vi "Main UI.vi"(11 "FormulaLV App in":refnum<class "FormulaG App.lvclass">) -> ()   [LabVIEW 2024, in "FormulaG.lvlib" / "FormulaG App.lvclass"]
uses:
  FormulaG App.lvclass
  FormulaG-Common/Camera.ctl
  <vilib>/sklein/WebView2/Webview2 Control/WebView2 Control.xctl
  UI State.ctl
  FormulaG App.lvclass/FormulaG App.ctl
  FormulaG-Common/UI Options.ctl
  State Update.ctl
  FormulaG-Common/Car State.ctl
  FormulaG-Common/Ranges.ctl
  FormulaG-Common/Car Info.ctl
  FormulaG-Common/Car Control.ctl
  FormulaG-Common/FormulaG-Common.lvlib
  FormulaG API/FormulaG API.lvclass
  <vilib>/IlluminatedG/IG GodotServer/GodotLV/GodotServer/GodotServer.lvclass
  Pause Cmd/Pause Cmd.lvclass
  Select Cam Cmd/Select Cam Cmd.lvclass
  UI Options Cmd/UI Options Cmd.lvclass
  Reset Cmd/Reset Cmd.lvclass
  <vilib>/IlluminatedG/IG OBS API/obs-websocket/OBS/OBS.lvclass
panel:
  out "UI Cover":string="\n\n\n\n\n\n\n\n\n\n\n\n\n\n\n\n\nWaiting for connection to game engine..."
  out "Fastest Lap":i32
  out "Fastest Lap Time":dbl format="%<%M:%S%3u>t"
  out "Lap":u8
  out "Update Rate":dbl format="%.2f"
  out "Web":string(xcontrol)
  out "Throttle":sgl(slide) scale=0.0..1.0
  out "Speed":sgl(knob) scale=0.0..10.0
  in  "Clear Map":bool
  out "Last Lap":dbl format="%<%M:%S%3u>t"
  out "Current Lap":dbl format="%<%M:%S%3u>t"
  out "XY Graph":cluster{dbl[], dbl[]}[](graph)
  in  "Pause":bool
  out "Chart":dbl[][](graph)
  in  "Camera":T1
  in  "Reset":bool
  out "Steering":sgl(knob) scale=-1.0..1.0
  out "Connected":bool
  in  "Show Range Lines":bool
  # "Map"
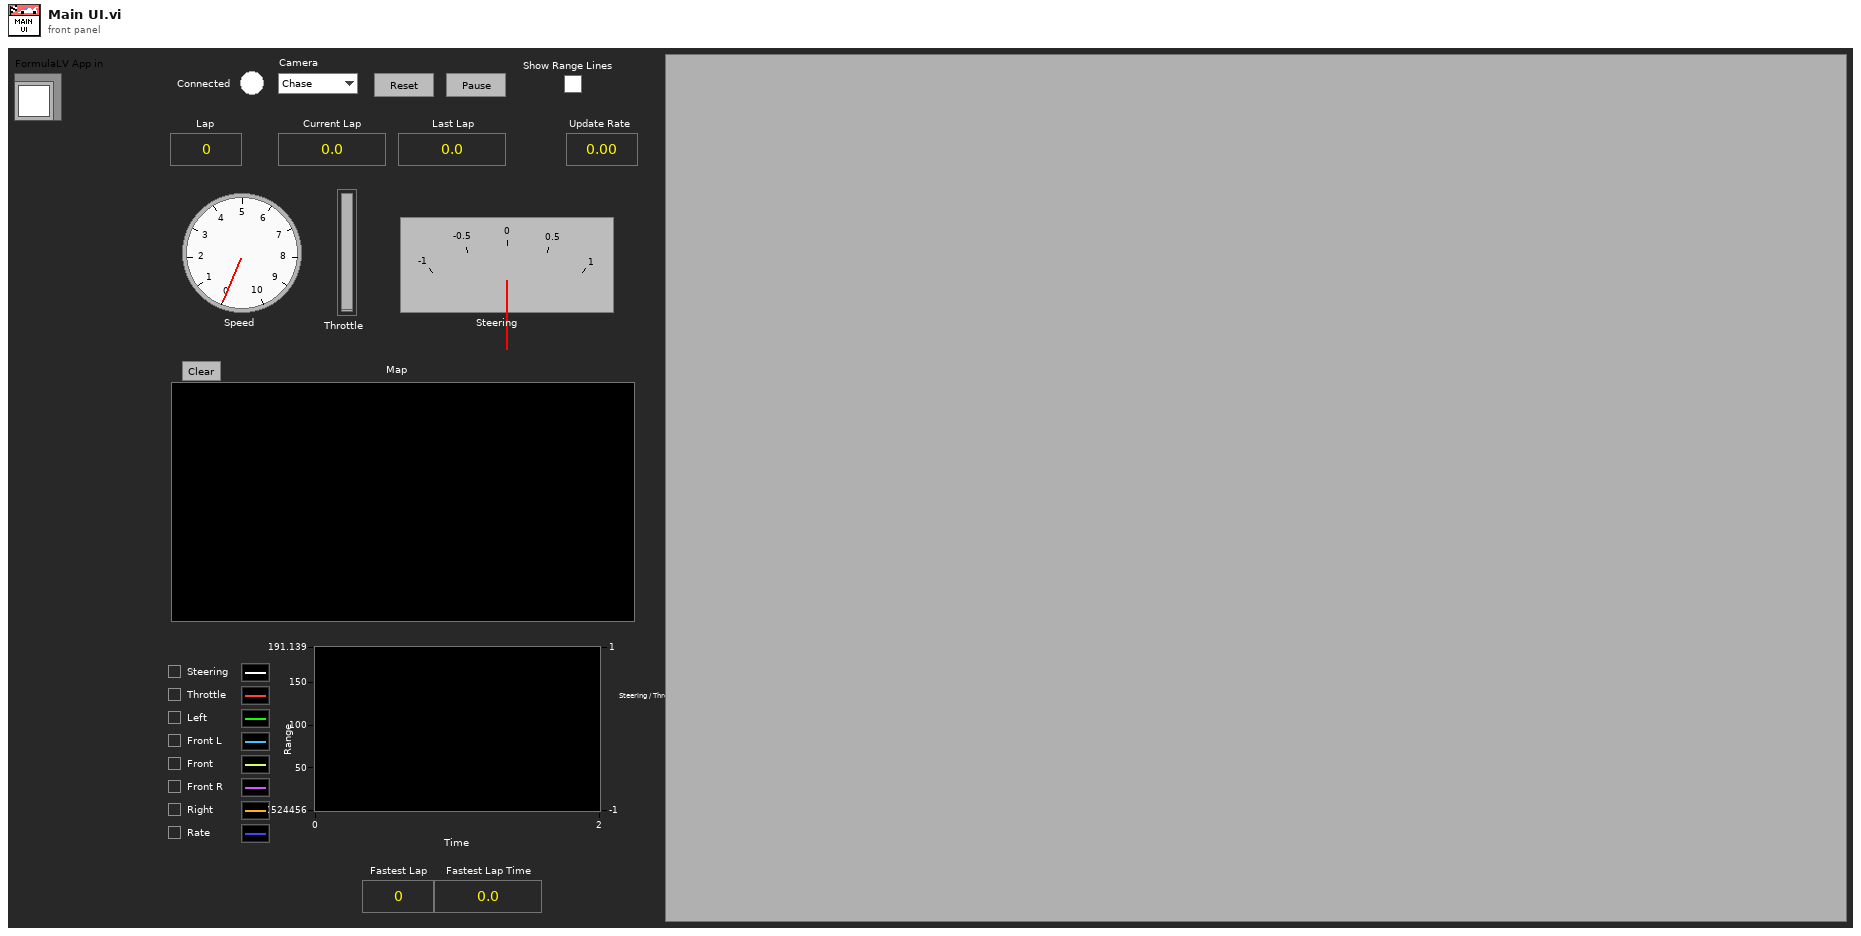
[diagram p1: front panel]
types:
  T1 = typedef "FormulaG-Common.lvlib/Camera.ctl" = enum16{"Chase", "Overhead"}
  T2 = typedef "FormulaG.lvlib/FormulaG App.lvclass/UI State.ctl" = enum16{"Init", "Connect", "Run", "Close"}
  T3 = typedef "FormulaG-Common.lvlib/UI Options.ctl" = cluster{"Range Visible":bool}
  T4 = typedef "LVRectTypeDef.ctl" = cluster{"Left":i16, "Top":i16, "Right":i16, "Bottom":i16}
  T5 = typedef "FormulaG-Common.lvlib/Car Control.ctl" = cluster{"Steering (-1 to 1)":sgl, "Throttle (0 to 1)":sgl}
  T6 = typedef "FormulaG-Common.lvlib/Car State.ctl" = cluster{"Ranges":T7, "Car Info":T8, "Current Lap":dbl, "Last Lap":dbl, "Lap":u8}
  T7 = typedef "FormulaG-Common.lvlib/Ranges.ctl" = cluster{"Front":sgl[], "Rear":sgl[]}
  T8 = typedef "FormulaG-Common.lvlib/Car Info.ctl" = cluster{"Speed":sgl, "X":sgl, "Y":sgl, "Heading":sgl}
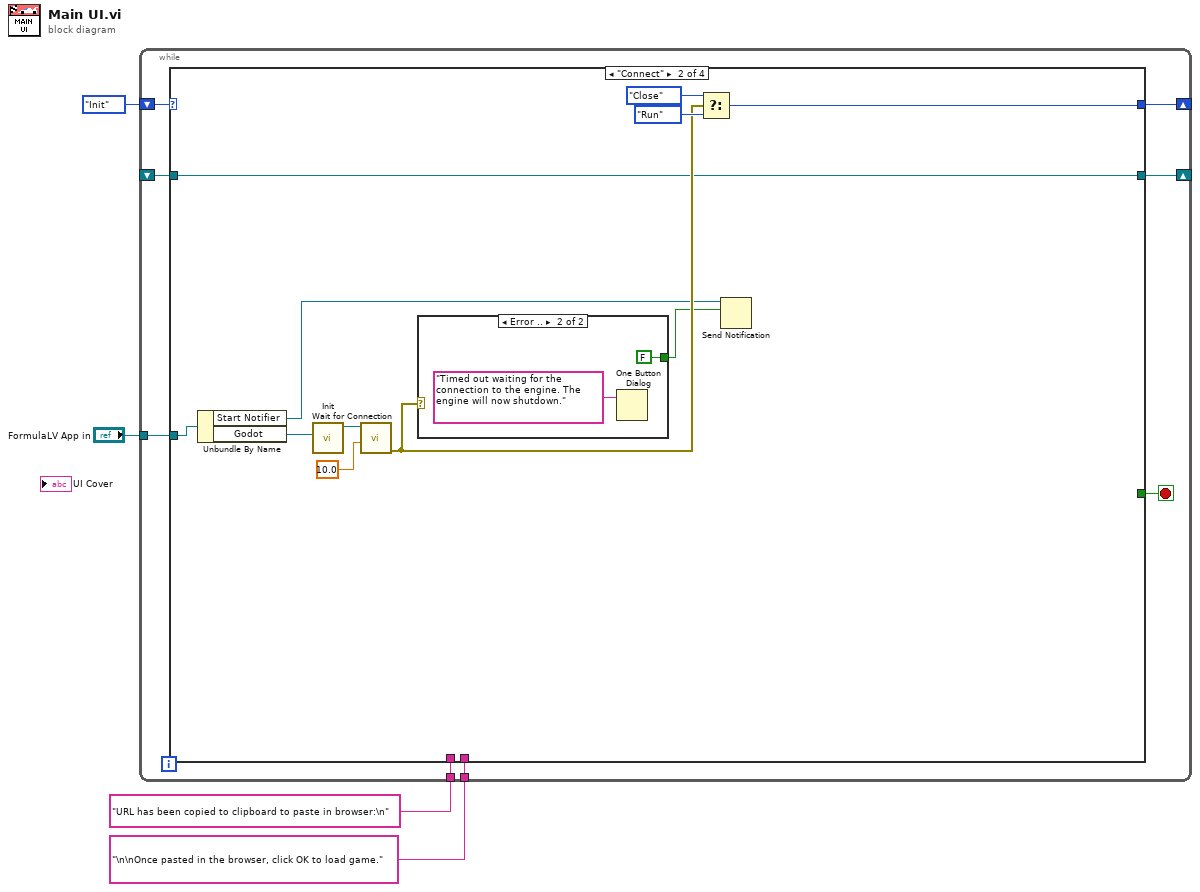
[diagram p0: block diagram]
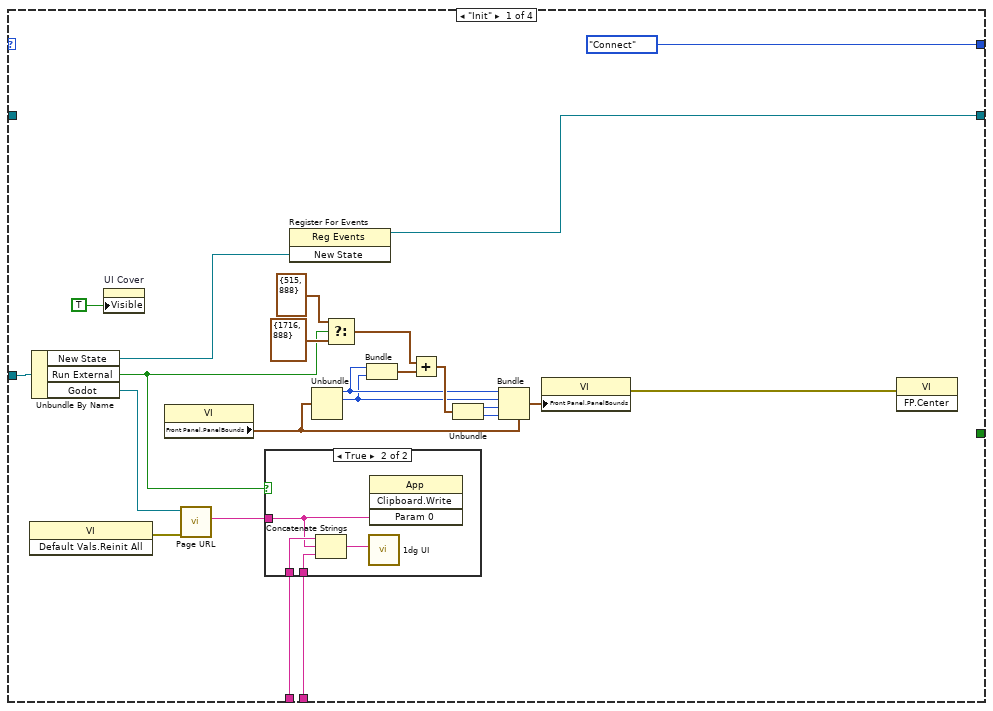
[diagram p2: hidden frame]
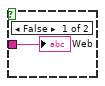
[diagram p3: hidden frame]
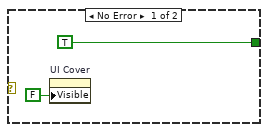
[diagram p4: hidden frame]
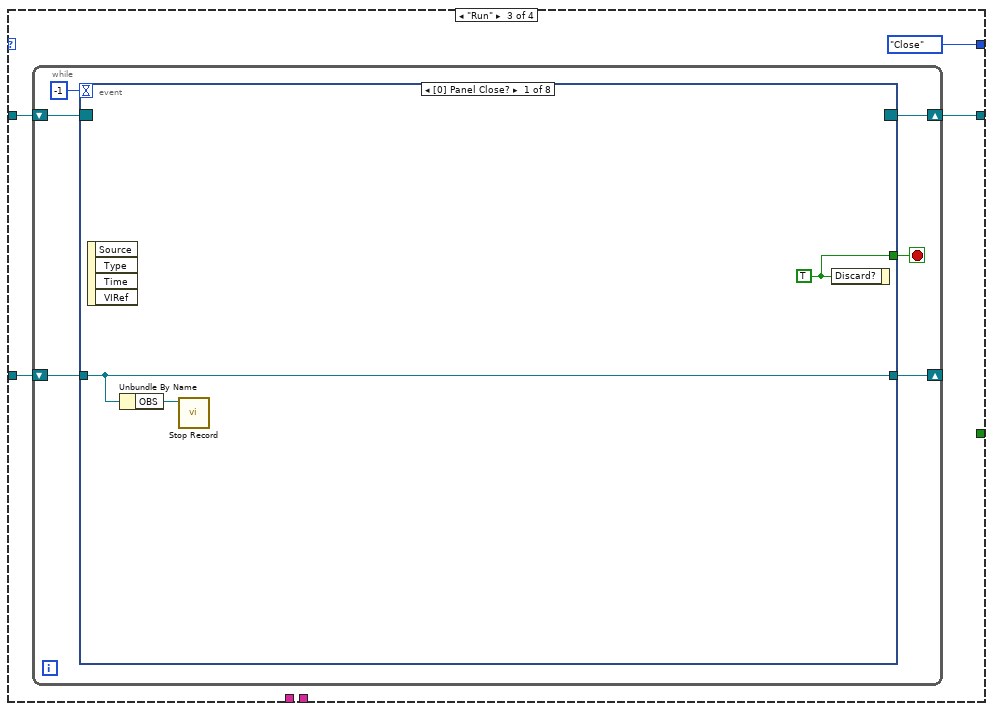
[diagram p5: hidden frame]
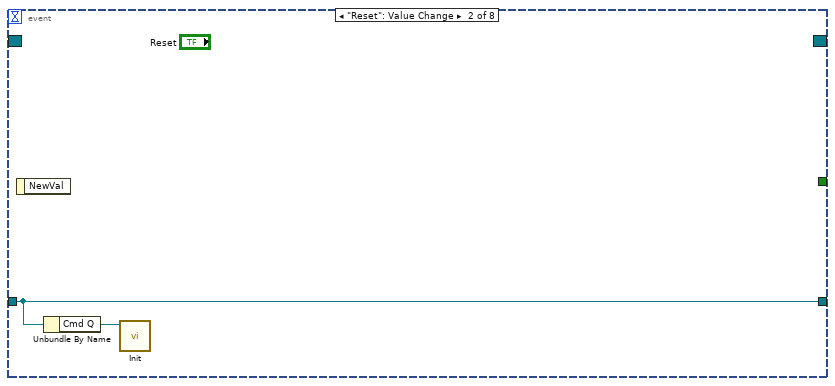
[diagram p6: hidden frame]
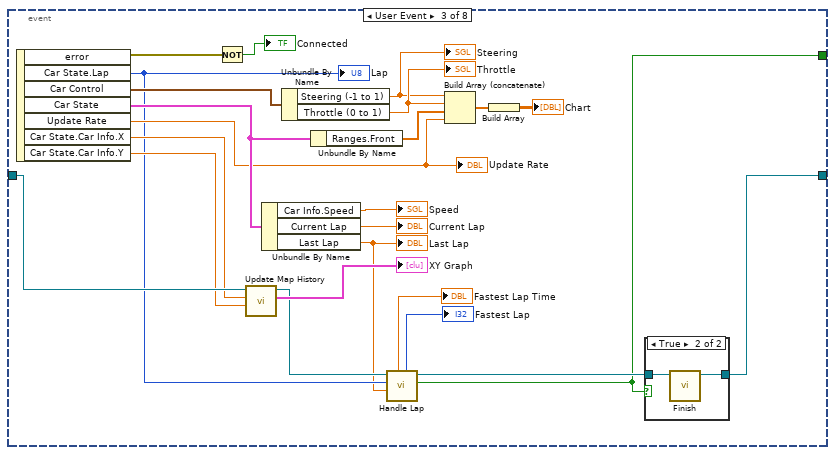
[diagram p7: hidden frame]
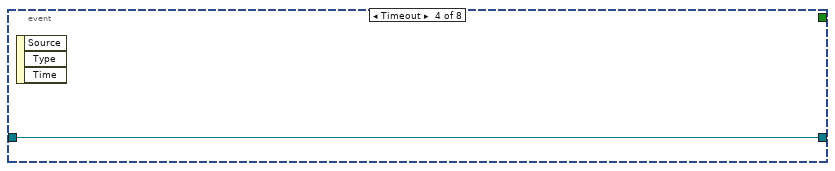
[diagram p9: hidden frame]
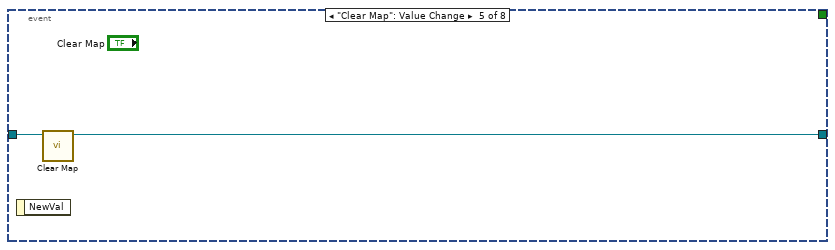
[diagram p10: hidden frame]
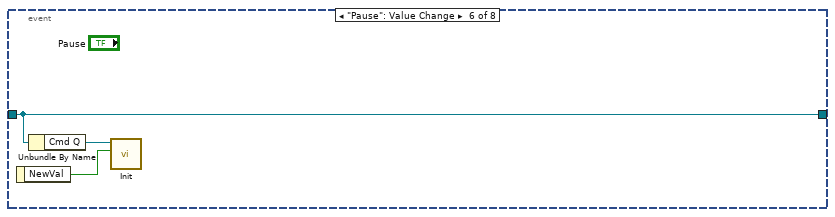
[diagram p11: hidden frame]
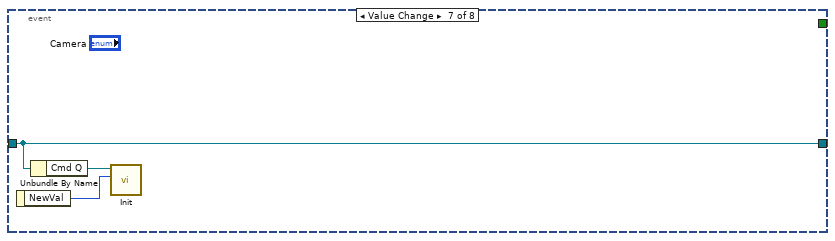
[diagram p12: hidden frame]
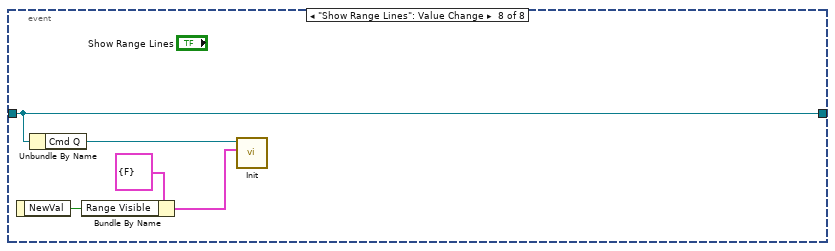
[diagram p13: hidden frame]
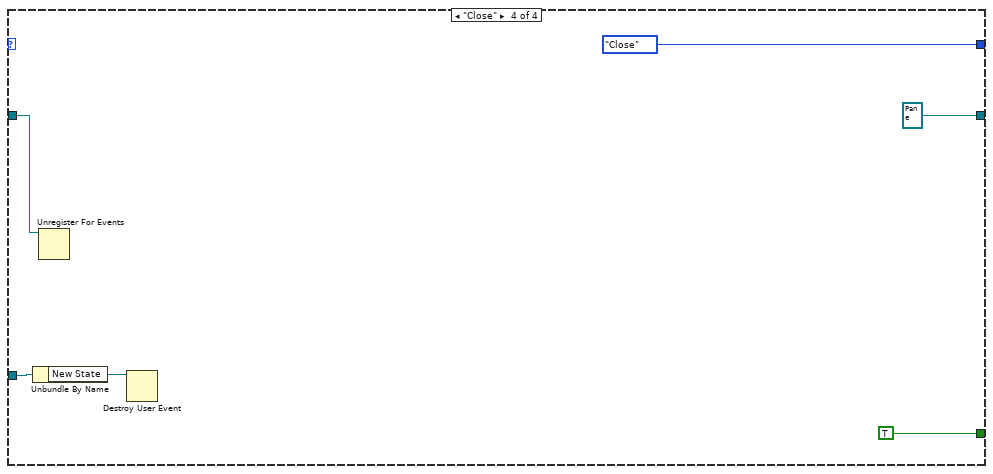
[diagram p14: hidden frame]
diagram:
  n1 = while {
    tunnel: "FormulaLV App in" -> [w12]
    shift-right: [w9] -> _
    shift-left: UI_State."Init" ("UI State") -> [w11]
    shift-right: [w8] -> _
    shift-left: _ -> [w7]
    tunnel: "URL has been copied to clipboard to paste in browser:\n" -> [w6]
    tunnel: "\n\nOnce pasted in the browser, click OK to load game." -> [w5]
    stop <- w10 stop-if-true
    n2 = case shown="\"Connect\"" w11 {
      tunnel: w12 -> [w32 w48 w59 w113]
      tunnel: [_ _ _ TRUE] -> w10
      tunnel: [UI_State."Connect" ("UI State") w51 UI_State."Close" ("UI State") UI_State."Close" ("UI State")] -> w9
      tunnel: [w28 w44 w56 refnum<event-registration> refnum ("Event Registration Refnum")] -> w8
      tunnel: w7 -> [_ w44 w57 w114]
      tunnel: w6 -> [w15 _ _ _]
      tunnel: w5 -> [w14 _ _ _]
      frame "Init" {
        n3 = invoke class="VI" method="Default Vals.Reinit All"() -> (error out=w35:errorcluster)  [unwired: 3 in, 2 out]
        n4 = Unbundle By Name(w32) -> ("New State"=w29:refnum<user-event>, "Run External"=w25:bool, "Godot"=w33:refnum<class "GodotServer.lvclass">)
        n5 = property on="UI Cover" class="Str"("Visible"=TRUE) -> ()  [unwired: 2 in, 2 out]
        n6 = property class="VI"() -> ("Front Panel.PanelBounds"=w23:T4)  [unwired: 2 in, 2 out]
        n7 = call <vilib>:"Page URL.vi"("error in (no error)"=w35, "GodotServer in"=w33) -> ("Page URL"=w34:string)  [unwired: 7 in, 2 out]
        n8 = case shown="True" w25 {
          tunnel: w34 -> [w36 w38]
          tunnel: w15 -> [_ w40]
          tunnel: w14 -> [_ w39]
          frame False {
            "Web" <- w36
          }
          frame True {
            n9 = Concatenate Strings(w40, w38, w39) -> (w37:string)
            n10 = call "1dg UI.vi"("String"=w37) -> ()  [unwired: 11 in]
            n11 = invoke class="App" method="Clipboard.Write"("Param 0"=w38) -> ()  [unwired: 3 in, 4 out]
          }
        }
        n12 = register-events(w29) -> (reference out=w28:refnum<event-registration>)  [unwired: 2 in, 1 out]
        n13 = Unbundle(w23) -> ("Left"=w17:i16, "Top"=w16:i16)  [unwired: 2 out]
        n14 = Select(t=cluster{i16, i16} {515, 888} ("External"), s=w25, f=cluster{i16, i16} {1716, 888} ("External")) -> (s? t:f=w21:cluster{i16, i16})
        n15 = Bundle("Left"=w17, "Top"=w16) -> (w24:cluster{"Left":i16, "Top":i16})  [unwired: 1 in]
        n16 = Add(x=w21, y=w24) -> (x+y=w20:cluster{i16, i16})
        n17 = Unbundle(w20) -> (w18:i16, w19:i16)
        n18 = Bundle(cluster=w23, "Left"=w17, "Top"=w16, "Right"=w18, "Bottom"=w19) -> (w22:T4)
        n19 = property class="VI"("Front Panel.PanelBounds"=w22) -> (error out=w13:errorcluster)  [unwired: 2 in, 1 out]
        n20 = invoke class="VI" method="FP.Center"(error in=w13) -> ()  [unwired: 2 in, 3 out]
      }
      frame "Connect" {
        n21 = Unbundle By Name(w48) -> ("Start Notifier"=w41:refnum<notifier>, "Godot"=w47:refnum<class "GodotServer.lvclass">)
        n22 = call "Init.vi"("Godot"=w47) -> ("FormulaG API out"=w46:refnum<class "FormulaG API.lvclass">)  [unwired: 9 in, 1 out]
        n23 = call "Wait for Connection.vi"("Timeout S (30)"=10.0, "FormulaG API in"=w46) -> ("error out"=w45:errorcluster)  [unwired: 7 in, 2 out]
        n24 = case shown="Error .." w45 {
          tunnel: [TRUE FALSE] -> w42
          frame No Error {
            n25 = property on="UI Cover" class="Str"("Visible"=FALSE) -> ()  [unwired: 2 in, 2 out]
          }
          frame Error {
            n26 = One Button Dialog(message="Timed out waiting for the connection to the engine. The engine will now shutdown.") -> ()  [unwired: 1 in, 1 out]
          }
        }
        n27 = Select(t=UI_State."Close" ("UI State"), s=w45, f=UI_State."Run" ("UI State")) -> (s? t:f=w51:T2)
        n28 = Send Notification(notification=w42, notifier=w41) -> ()  [unwired: 1 in, 2 out]
      }
      frame "Run" {
        n29 = while {
          shift-right: [w61] -> w56
          shift-left: w57 -> [w62]
          shift-right: [w60] -> _
          shift-left: w59 -> [w64]
          stop <- w65 stop-if-true
          n30 = event shown="[0] Panel Close?" {
            selector: w62 -> [_ _ _ _ _ _ _ _]
            dyn-events: [_ _ _ _ _ _ _ _] -> w61
            timeout: -1 -> [_ _ _ _ _ _ _ _]
            tunnel: [w68 _ w71 _ _ _ _ _] -> w65
            tunnel: w64 -> [w67 w70 w92 w98 w100 w103 w106 w111]
            tunnel: [w67 w70 w77 w98 w99 w103 w106 w111] -> w60
            event Panel Close? {
              w68 = TRUE ("Discard?")
              n31 = event-data() -> ()  [unwired: 1 in, 4 out]
              n32 = Unbundle By Name(w67) -> ("OBS"=w66:refnum<class "OBS.lvclass">)
              n33 = call <vilib>:"Stop Record.vi"("OBS in"=w66) -> ()  [unwired: 8 in, 3 out]
              n34 = event-data("Discard?"=w68) -> ()  [unwired: 1 in, 1 out]
            }
            event "Reset": Value Change {
              n35 = event-data() -> ()  [unwired: 1 in, 1 out]
              n36 = Unbundle By Name(w70) -> ("Cmd Q"=w69:refnum<queue>)
              n37 = call "Init.vi"("Cmd Q"=w69) -> ()  [unwired: 11 in]
            }
            event User Event {
              n38 = event-data() -> ("error"=w80:errorcluster, "Car State.Lap"=w75:u8, "Car Control"=w88:T5, "Car State"=w84:T6, "Update Rate"=w81:dbl, "Car State.Car Info.X"=w91:sgl, "Car State.Car Info.Y"=w90:sgl)  [unwired: 1 in]
              "Update Rate" <- w81
              "Lap" <- w75
              n39 = Not(x=w80) -> (.not. x?=→"Connected":bool)
              n40 = call "Update Map History.vi"("Y"=w90, "X"=w91, "FormulaG App in"=w92) -> ("XY Graph"=→"XY Graph":cluster{dbl[], dbl[]}[], "FormulaG App out"=w78:refnum<class "FormulaG App.lvclass">)  [unwired: 6 in, 1 out]
              n41 = Unbundle By Name(w84) -> ("Car Info.Speed"=→"Speed":sgl, "Current Lap"=→"Current Lap":dbl, "Last Lap"=w74:dbl)
              "Last Lap" <- w74
              n42 = Unbundle By Name(w88) -> ("Steering (-1 to 1)"=w82:sgl, "Throttle (0 to 1)"=w83:sgl)
              "Steering" <- w82
              "Throttle" <- w83
              n43 = Unbundle By Name(w84) -> ("Ranges.Front"=w87:sgl[])
              n44 = call "Handle Lap.vi"("Last Lap"=w74, "Lap"=w75, "FormulaG App in"=w78) -> ("Finish"=w71:bool, "FormulaG App out"=w76:refnum<class "FormulaG App.lvclass">, "Fastest Lap"=→"Fastest Lap":i32, "Min Time"=→"Fastest Lap Time":dbl)  [unwired: 4 in, 1 out]
              n45 = Build Array (concatenate)(w82, w83, w87, w81) -> (w86:dbl[])
              n46 = Build Array(w86) -> (→"Chart":dbl[][])
              n47 = case shown="True" w71 {
                tunnel: w76 -> [w95 w97]
                tunnel: [w95 w96] -> w77
                frame False {
                }
                frame True {
                  n48 = call "Finish.vi"("FormulaG App in"=w97) -> ("FormulaG App out"=w96:refnum<class "FormulaG App.lvclass">)  [unwired: 9 in, 1 out]
                }
              }
            }
            event Timeout {
              n49 = event-data() -> ()  [unwired: 1 in, 3 out]
            }
            event "Clear Map": Value Change {
              n50 = event-data() -> ()  [unwired: 1 in, 1 out]
              n51 = call "Clear Map.vi"("FormulaG App in"=w100) -> ("FormulaG App out"=w99:refnum<class "FormulaG App.lvclass">)  [unwired: 9 in, 1 out]
            }
            event "Pause": Value Change {
              n52 = event-data() -> ("NewVal"=w102:bool)  [unwired: 1 in]
              n53 = Unbundle By Name(w103) -> ("Cmd Q"=w101:refnum<queue>)
              n54 = call "Init.vi"("Pause"=w102, "Cmd Q"=w101) -> ()  [unwired: 9 in, 1 out]
            }
            event Value Change {
              n55 = event-data() -> ("NewVal"=w105:T1)  [unwired: 1 in]
              n56 = Unbundle By Name(w106) -> ("Cmd Q"=w104:refnum<queue>)
              n57 = call "Init.vi"("Camera"=w105, "Cmd Q"=w104) -> ()  [unwired: 9 in, 1 out]
            }
            event "Show Range Lines": Value Change {
              n58 = event-data() -> ("NewVal"=w109:bool)  [unwired: 1 in]
              n59 = Unbundle By Name(w111) -> ("Cmd Q"=w108:refnum<queue>)
              n60 = Bundle By Name(cluster=T3 {"Range Visible"=FALSE} ("UI Options"), "Range Visible"=w109) -> (w107:T3)
              n61 = call "Init.vi"("UI Options"=w107, "Cmd Q"=w108) -> ()  [unwired: 9 in, 1 out]
            }
          }
        }
      }
      frame "Close" {
        n62 = Unbundle By Name(w113) -> ("New State"=w112:refnum<user-event>)
        n63 = Unregister For Events(event registration refnum=w114) -> ()  [unwired: 1 in, 1 out]
        n64 = Destroy User Event(user event=w112) -> ()  [unwired: 1 in, 1 out]
      }
    }
  }
